vi "Set Desaccading Parameters.vi"(8 "error in (no error)":errorcluster, 10 "Parameter":T1={"Threshold 1 [Acc]"=0.0, "Threshold 2 [% of TH1]"=0, "tolerance"=2.0, "Search WD "=0.05757575757575758, " always use TH2"=TRUE, "SD for Outliers"=3.0303030303030303, "Max time [ms]"=50.0, "Min time [ms]"=1.0, "Velocity Threshold"=0.05757575757575758} {"Velocity Threshold" scale=50.0..400.0; "SD for Outliers" scale=0.0..5.0; "Search WD" scale=0.0..0.3; "tolerance" scale=0.0..100.0; "Threshold 2 [% of TH1]" scale=0.0..100.0; "Threshold 1 [Acc]" scale=1.0..40000.0}, 11 "Desaccade Manipulator in":refnum<class "Desaccade Manipulator.lvclass">) -> (0 "error out":errorcluster, 3 "Desaccade Manipulator out":refnum<class "Desaccade Manipulator.lvclass">)   [LabVIEW 2016, in "Desaccade Manipulator.lvclass"]
uses:
  Desaccade Manipulator.lvclass
  Typedef - Desaccading Parameter.ctl
  Desaccade Manipulator.lvclass/Desaccade Manipulator.ctl
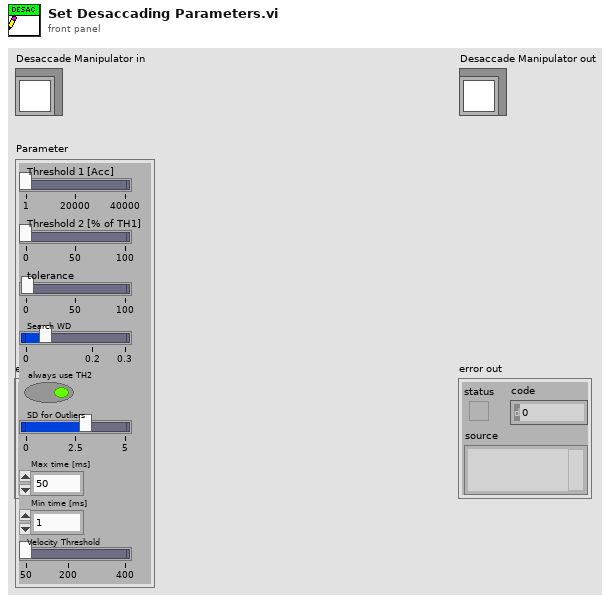
[diagram p1: front panel]
types:
  T1 = typedef "Typedef - Desaccading Parameter.ctl" = cluster{"Threshold 1 [Acc]":dbl, "Threshold 2 [% of TH1]":i32, "tolerance":dbl, "Search WD ":dbl, " always use TH2":bool, "SD for Outliers":dbl, "Max time [ms]":dbl, "Min time [ms]":dbl, "Velocity Threshold":dbl}
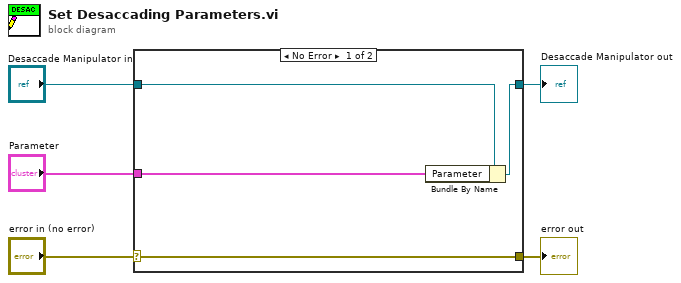
[diagram p0: block diagram]
diagram:
  n1 = case shown="No Error" "error in (no error)" {
    selector: "error in (no error)" -> [w9 w10]
    tunnel: [w9 w10] -> w4
    tunnel: [w7 w11] -> w2
    tunnel: "Desaccade Manipulator in" -> [w8 w11]
    tunnel: "Parameter" -> [w6 _]
    frame No Error {
      n2 = Bundle By Name(cluster=w8, "Parameter"=w6) -> (w7:refnum<class "Desaccade Manipulator.lvclass">)
    }
    frame Error {
    }
  }
  "error out" <- w4
  "Desaccade Manipulator out" <- w2
